vi "Set Up Create New.vi"(8 "error in (no error)":errorcluster, 11 "Test Case in":refnum<class "Routing and Faulting Import Unit Tests.lvclass">) -> (0 "error out":errorcluster, 1 "Import Path":path, 2 "Routing and Faulting Custom Device Ref":T1=18446744073709551615 format="%.0x", 3 "Test Case out":refnum<class "Routing and Faulting Import Unit Tests.lvclass">)   [LabVIEW 2020, in "Routing and Faulting Import Unit Tests.lvclass"]
uses:
  Routing and Faulting Import Unit Tests.lvclass
  <vilib>/NI VeriStand/Custom Device API/Custom Device Item Ref.ctl
  Routing and Faulting Import Unit Tests.lvclass/Routing and Faulting Import Unit Tests.ctl
  <userlib>/_OpenG.lib/file/file.llb/Append Path to Root if Relative - Scalar__ogtk.vi
  Scripting/Routing and Faulting Scripting.lvlib
  niveristand-custom-device-testing-tools/VeriStandTestUtilities/VeriStandTestUtilities.lvlib
  <vilib>/NI VeriStand/Custom Device API/Custom Device API.lvlib
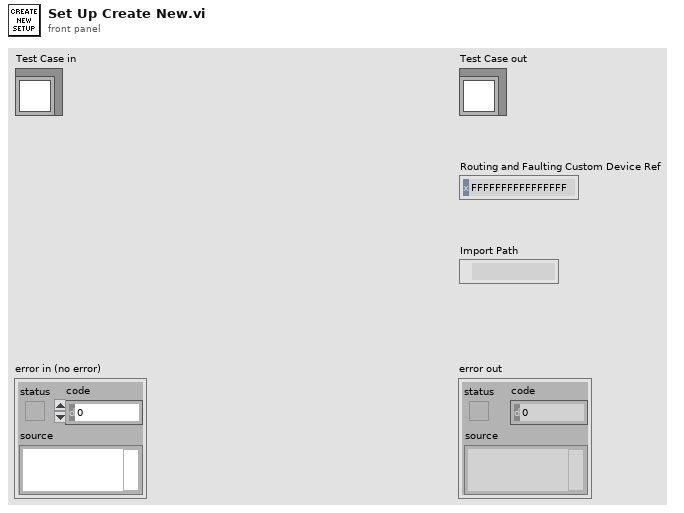
[diagram p1: front panel]
types:
  T1 = typedef "Custom Device API.lvlib/Custom Device Item Ref.ctl" = u64
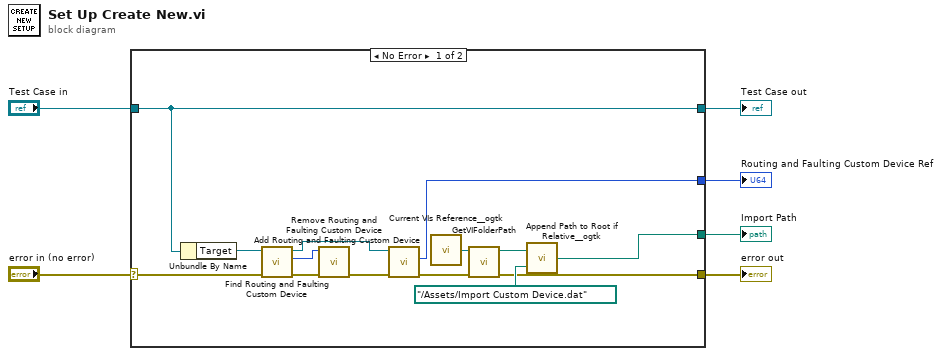
[diagram p0: block diagram]
diagram:
  n1 = case shown="No Error" "error in (no error)" {
    selector: "error in (no error)" -> [w11 w22]
    tunnel: [w8 w22] -> w5
    tunnel: [w10 w21] -> w3
    tunnel: "Test Case in" -> [w10 w21]
    tunnel: [w9 _] -> w2
    tunnel: [w7 _] -> w1
    frame No Error {
      n2 = Unbundle By Name(w10) -> ("Target"=w12:refnum<k24>)
      n3 = call "Find Routing and Faulting Custom Device.vi"("error in"=w11, "target in"=w12) -> ("error out"=w16:errorcluster, "routing and faulting custom device"=w15:T1, "target out"=w14:refnum<k24>)  [unwired: 7 in]
      n4 = call "Remove Routing and Faulting Custom Device.vi"("error in"=w16, "routing and faulting custom device"=w15) -> ("error out"=w13:errorcluster)  [unwired: 9 in]
      n5 = call "Add Routing and Faulting Custom Device.vi"("error in"=w13, "target in"=w14) -> ("error out"=w20:errorcluster, "routing and faulting custom device"=w9:T1)  [unwired: 7 in, 1 out]
      n6 = call <userlib>:"Current VIs Reference__ogtk.vi"() -> ("Current VI's reference"=w19:refnum<vi>)  [unwired: 5 in]
      n7 = call "GetVIFolderPath.vi"("error in (no error)"=w20, "VI Reference in"=w19) -> ("error out"=w8:errorcluster, "VI Folder Path out"=w18:path)  [unwired: 8 in]
      n8 = call-poly <userlib>:"Append Path to Root if Relative__ogtk.vi"("Absolute or Relative Path"=path "../Assets/Import Custom Device.dat", "Root Path"=w18) -> ("Absolute or Appended Path"=w7:path)
    }
    frame Error {
    }
  }
  "error out" <- w5
  "Test Case out" <- w3
  "Routing and Faulting Custom Device Ref" <- w2
  "Import Path" <- w1
